vi "Next Available Datum Index Ranges.vi"(0 "bytestream":refnum<class "Bytestream.lvclass">, 1 "length":i32) -> (4 "start":i32, 5 "initial length":i32, 6 "terminal length":i32)   [LabVIEW 2020, in "NI_Bytestream.lvlib" / "Bytestream.lvclass"]
uses:
  <vilib>/Array/Bytestream/Bytestream.lvclass
  <vilib>/Array/Bytestream/Bytestream.lvclass/Bytestream.ctl
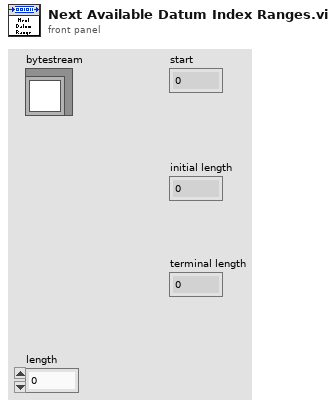
[diagram p1: front panel]
types:
  T1 = typedef "NI_Bytestream.lvlib/Bytestream.lvclass/Datum.ctl" = cluster{"array":u8[], "index":i32}
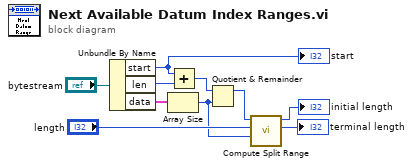
[diagram p0: block diagram]
diagram:
  n1 = Unbundle By Name("bytestream") -> ("start"=w9:i32, "len"=w8:i32, "data"=w7:T1[])
  "start" <- w9
  n2 = Array Size(array=w7) -> (size(s)=w3:i32)
  n3 = Add(x=w9, y=w8) -> (x+y=w6:i32)
  n4 = Quotient & Remainder(x=w6, y=w3) -> (x-y*floor(x/y)=w5:i32)  [unwired: 1 out]
  n5 = call <vilib>:"Compute Split Range.vi"("limit size"=w3, "length"="length", "start"=w5) -> ("terminal length"=→"terminal length":i32, "initial length"=→"initial length":i32)  [unwired: 7 in]
